vi "Tiny_Script_Packets.vi"(2 "Lines in":string[](array[string]), 3 "Max Size":i32=500, 4 "Execution Mode":T1(ring)=enum."Load and Run") -> (0 "# chars":i32, 1 "Lines of Script":string[](array[string]))   [LabVIEW 2012]
uses:
  <userlib>/botspeak/VIs/SubVIs/BotSpeak_Globals.vi
panel:
  out "# lines":i32
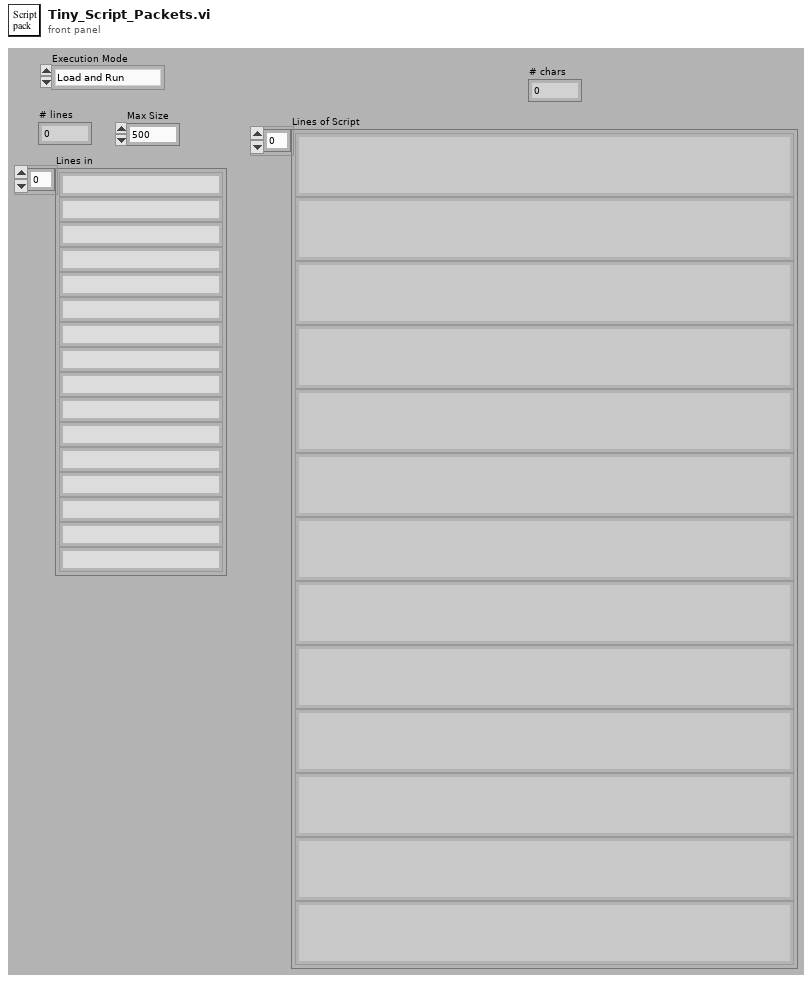
[diagram p1: front panel]
types:
  T1 = enum16{"Load", "Run", "Load and Run", "Debug, Run", "Run, Wait"}
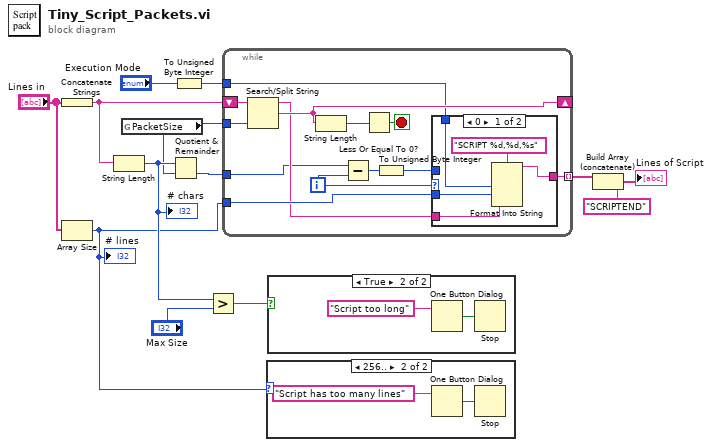
[diagram p0: block diagram]
diagram:
  n1 = Concatenate Strings("Lines in") -> (w10:string)
  n2 = Array Size(array="Lines in") -> (size(s)=w5:i32)
  "# lines" <- w5
  n3 = String Length(string=w10) -> (length=w12:i32)
  "# chars" <- w12
  n4 = global read "BotSpeak_Globals.vi" "PacketSize"() -> (w1:i32)
  n5 = Quotient & Remainder(x=w12, y=w1) -> (floor(x/y)=w13:i32)  [unwired: 1 out]
  n6 = To Unsigned Byte Integer(number="Execution Mode") -> (unsigned 8bit integer=w11:u8)
  n7 = Greater?(x=w12, y="Max Size") -> (0:w8:bool)
  n8 = while {
    shift-right: [w25] -> _
    shift-left: w10 -> [w26]
    tunnel: [w20] -> w4 mode=indexing
    tunnel: w11 -> [w16]
    tunnel: w5 -> [w22]
    tunnel: w1 -> [w19]
    tunnel: w13 -> [w18]
    i -> [w15]
    stop <- w23 stop-if-true
    n9 = Search/Split String(string=w26, offset (0)=w19) -> (substring before match=w21:string, match + rest of string=w25:string)  [unwired: 1 in, 1 out]
    n10 = String Length(string=w25) -> (length=w24:i32)
    n11 = Subtract(x=w18, y=w15) -> (x-y=w17:i32)
    n12 = Less Or Equal To 0?(x=w24) -> (x <= 0?=w23:bool)
    n13 = To Unsigned Byte Integer(number=w17) -> (unsigned 8bit integer=w14:u8)
    n14 = case shown="0" w15 {
      tunnel: w22 -> [w30 _]
      tunnel: w21 -> [w29 w32]
      tunnel: [w28 w32] -> w20
      tunnel: w16 -> [w27 _]
      tunnel: w14 -> [_ _]
      frame 0 {
        n15 = Format Into String(format string="SCRIPT %d,%d,%s" ("command"), w27, w30, w29) -> (resulting string=w28:string)  [unwired: 2 in, 1 out]
      }
      frame Default {
      }
    }
  }
  n16 = case shown="256.." w5 {
    frame ..255 {
    }
    frame 256.. {
      n17 = One Button Dialog(message="Script has too many lines" ("command")) -> (true=w33:bool)  [unwired: 1 in]
      n18 = Stop(stop? (T)=w33) -> ()
    }
  }
  n19 = case shown="True" w8 {
    frame False {
    }
    frame True {
      n20 = One Button Dialog(message="Script too long" ("command")) -> (true=w35:bool)  [unwired: 1 in]
      n21 = Stop(stop? (T)=w35) -> ()
    }
  }
  n22 = Build Array (concatenate)(w4, "SCRIPTEND" ("command")) -> (→"Lines of Script":string[])
